vi "Sort data for upload.vi"(7 "Add reset (T)":bool=TRUE, 9 "Colour array in":u32[](array[numeric]), 10 "Zero Outputs?":bool, 11 "ID":u32) -> (3 "Upload data":u32[](array[numeric]))   [LabVIEW 2025]
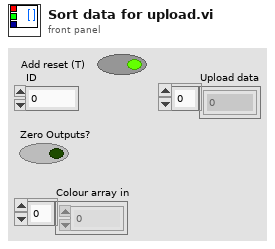
[diagram p1: front panel]
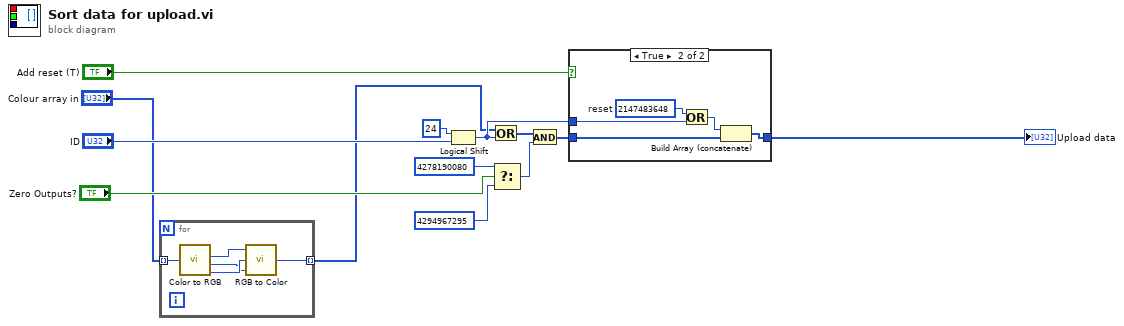
[diagram p0: block diagram]
diagram:
  n1 = for {
    tunnel: "Colour array in" -> [w18] mode=indexing
    tunnel: [w17] -> w1 mode=indexing
    n2 = call <vilib>:"Color to RGB.vi"("Color"=w18) -> ("R"=w16:u8, "G"=w14:u8, "B"=w15:u8)  [unwired: 1 out]
    n3 = call <vilib>:"RGB to Color.vi"("B"=w14, "G"=w15, "R"=w16) -> ("Color"=w17:u32)
  }
  n4 = Logical Shift(y=i16 24, x="ID") -> (x << y=w3:u32)
  n5 = Or(x=w1, y=w3) -> (x .or. y?=w13:u32[])
  n6 = Select(t=u32 4278190080, s="Zero Outputs?", f=u32 4294967295) -> (s? t:f=w9:u32)
  n7 = And(x=w13, y=w9) -> (x .and. y?=w8:u32[])
  n8 = case shown="True" "Add reset (T)" {
    tunnel: w8 -> [w19 w24]
    tunnel: [w19 w23] -> w7
    tunnel: w3 -> [_ w21]
    frame False {
    }
    frame True {
      w20 = u32 2147483648  # reset
      n9 = Or(x=w20, y=w21) -> (x .or. y?=w22:u32)
      n10 = Build Array (concatenate)(w22, w24) -> (w23:u32[])
    }
  }
  "Upload data" <- w7
